vi "ep_Write Inf File.vi"(8 "error in":errorcluster, 10 "inf content":string, 11 "task in":T1={"file refnums"=[], "Data Object"=refnum, "config info"={"station_name"="", "rec_dev_id"="", "rev_year"=1999.0, "TT"=0, "##A"=0, "##D"=0, "analog channel info"=[], "status channel info"=[], "lf"=-inf, "nrates"=65535, "samp info"=[], "initial timestamp"=timestamp(0 s since 1904-01-01), "trigger timestamp"=timestamp(0 s since 1904-01-01), "ft"=enum."Binary", "timemult"=1.0}, "public inf content"={"Source"="", "Record Type"=enum."Fault", "Phase ID"="", "Event Description"="", "Device ID"="", "Distance of Fault"=-1.0, "Distance Unit"=enum."Miles", "Max_Current"=inf, "Min_Current"=-inf, "Max_Voltage"=inf, "Min_Voltage"=-inf, "EventNoteCount"=0, "Event Information"=[]}, "private inf content"=[], "internal buffers"={"start index"=1, "config to public inf"=enum."disabled", "static config info"="", "static file_des record inf"="", "static file_des channel inf"="", "public inf"="", "private inf"=""}} {"public inf content"."Event Information"."min sample number" max=9999999999; "public inf content"."Event Information"."max sample number" max=9999999999; "config info"."nrates" max=999; "config info"."status channel info"."Dn" min=1 max=999999; "config info"."analog channel info"."An" min=1 max=999999; "config info"."trigger timestamp" format="%<%H:%M:%S%6u\n%d/%m/%Y>T"; "config info"."initial timestamp" format="%<%H:%M:%S%6u\n%d/%m/%Y>T"; "config info"."##D" max=999999; "config info"."##A" max=999999; "config info"."TT" min=1 max=999999; "config info"."rev_year" min=1999.0 max=1999.0}) -> (0 "error out":errorcluster, 3 "dup task":T1={"file refnums"=[], "Data Object"=refnum, "config info"={"station_name"="", "rec_dev_id"="", "rev_year"=1999.0, "TT"=0, "##A"=0, "##D"=0, "analog channel info"=[], "status channel info"=[], "lf"=-inf, "nrates"=65535, "samp info"=[], "initial timestamp"=timestamp(0 s since 1904-01-01), "trigger timestamp"=timestamp(0 s since 1904-01-01), "ft"=enum."Binary", "timemult"=1.0}, "public inf content"={"Source"="", "Record Type"=enum."Fault", "Phase ID"="", "Event Description"="", "Device ID"="", "Distance of Fault"=-1.0, "Distance Unit"=enum."Miles", "Max_Current"=inf, "Min_Current"=-inf, "Max_Voltage"=inf, "Min_Voltage"=-inf, "EventNoteCount"=0, "Event Information"=[]}, "private inf content"=[], "internal buffers"={"start index"=1, "config to public inf"=enum."disabled", "static config info"="", "static file_des record inf"="", "static file_des channel inf"="", "public inf"="", "private inf"=""}} {"public inf content"."Event Information"."min sample number" max=9999999999; "public inf content"."Event Information"."max sample number" max=9999999999; "config info"."nrates" max=999; "config info"."status channel info"."Dn" min=1 max=999999; "config info"."analog channel info"."An" min=1 max=999999; "config info"."trigger timestamp" format="%<%H:%M:%S%6u\n%d/%m/%Y>T"; "config info"."initial timestamp" format="%<%H:%M:%S%6u\n%d/%m/%Y>T"; "config info"."##D" max=999999; "config info"."##A" max=999999; "config info"."TT" min=1 max=999999; "config info"."rev_year" min=1999.0 max=1999.0})   [LabVIEW 2011, in "NI_EP_COMTRADE.lvlib"]
uses:
  <vilib>/addons/Electrical Power/File IO/NI_EP_COMTRADE.lvlib
  <vilib>/addons/Electrical Power/File IO/COMTRADE/typedefs/ep_Task.ctl
  <vilib>/addons/Electrical Power/File IO/COMTRADE/typedefs/ep_Config Info.ctl
  <vilib>/addons/Electrical Power/File IO/COMTRADE/typedefs/ep_Analog Channel Info.ctl
  <vilib>/addons/Electrical Power/File IO/COMTRADE/typedefs/ep_Status Channel Info.ctl
  <vilib>/addons/Electrical Power/File IO/COMTRADE/typedefs/ep_File Format.ctl
  <vilib>/addons/Electrical Power/File IO/COMTRADE/typedefs/ep_Public Inf Content.ctl
  <vilib>/addons/Electrical Power/File IO/COMTRADE/typedefs/ep_Public Event Inf.ctl
  <vilib>/addons/Electrical Power/File IO/COMTRADE/typedefs/ep_Private Inf Content.ctl
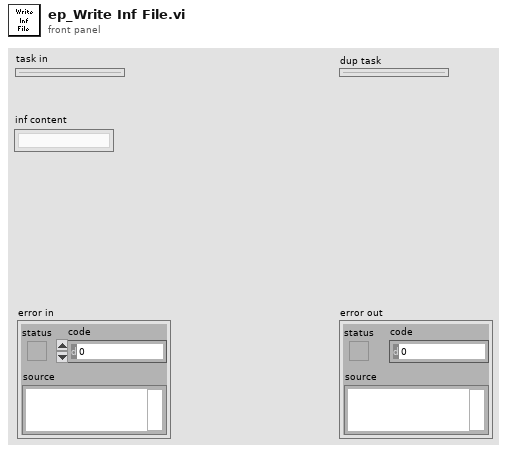
[diagram p1: front panel]
types:
  T1 = typedef "NI_EP_COMTRADE.lvlib/ep_Task.ctl" = cluster{"file refnums":refnum<file>[], "Data Object":refnum<k20>, "config info":T2, "public inf content":T6, "private inf content":T8, "internal buffers":cluster{"start index":u32, "config to public inf":enum16{"disabled", "enabled", "buffered"}, "static config info":string, "static file_des record inf":string, "static file_des channel inf":string, "public inf":string, "private inf":string}}
  T2 = typedef "NI_EP_COMTRADE.lvlib/ep_Config Info.ctl" = cluster{"station_name":string, "rec_dev_id":string, "rev_year":dbl, "TT":u32, "##A":u32, "##D":u32, "analog channel info":T3[], "status channel info":T4[], "lf":sgl, "nrates":u16, "samp info":cluster{"samp":sgl, "endsamp":u32}[], "initial timestamp":timestamp, "trigger timestamp":timestamp, "ft":T5, "timemult":sgl}
  T3 = typedef "NI_EP_COMTRADE.lvlib/ep_Analog Channel Info.ctl" = cluster{"An":u32, "ch_id":string, "ph":string, "ccbm":string, "uu":string, "a":sgl, "b":sgl, "skew":sgl, "min":i32, "max":i32, "primary":sgl, "secondary":sgl, "PS":enum16{"P", "S"}}
  T4 = typedef "NI_EP_COMTRADE.lvlib/ep_Status Channel Info.ctl" = cluster{"Dn":u32, "ch_id":string, "ph":string, "ccbm":string, "Y":bool}
  T5 = typedef "NI_EP_COMTRADE.lvlib/ep_File Format.ctl" = enum16{"ASCII", "Binary"}
  T6 = typedef "NI_EP_COMTRADE.lvlib/ep_Public Inf Content.ctl" = cluster{"Source":string, "Record Type":enum16{"Fault", "Unknown", "Misoperation", "Close", "Trip", "Reclose", "Power swing", "Simulation"}, "Phase ID":string, "Event Description":string, "Device ID":string, "Distance of Fault":dbl, "Distance Unit":enum16{"Miles", "Kilometers", "Percent of line", "Percent of setting", "Ohms"}, "Max_Current":dbl, "Min_Current":dbl, "Max_Voltage":dbl, "Min_Voltage":dbl, "EventNoteCount":u32, "Event Information":T7[]}
  T7 = typedef "NI_EP_COMTRADE.lvlib/ep_Public Event Inf.ctl" = cluster{"channel number":u32, "max value":dbl, "min value":dbl, "max sample number":u64, "min sample number":u64, "max sample text":string[], "min sample text":string[]}
  T8 = typedef "NI_EP_COMTRADE.lvlib/ep_Private Inf Content.ctl" = cluster{"Section Header":string, "Entry Names":string[], "Entry Values":string[]}[]
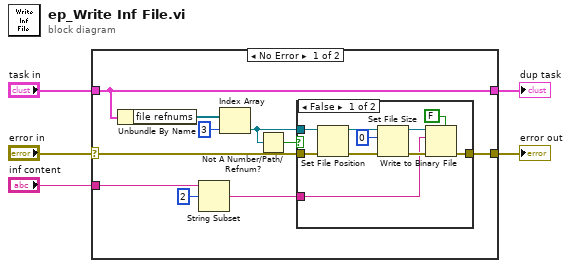
[diagram p0: block diagram]
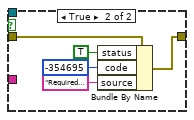
[diagram p2: hidden frame]
diagram:
  n1 = case shown="No Error" "error in" {
    selector: "error in" -> [w12 w31]
    tunnel: "task in" -> [w13 w32]
    tunnel: [w13 w32] -> w3
    tunnel: [w11 w31] -> w2
    tunnel: "inf content" -> [w10 _]
    frame No Error {
      n2 = Unbundle By Name(w13) -> ("file refnums"=w15:refnum<file>[])
      n3 = String Subset(string=w10, offset (0)=2) -> (substring=w6:string)  [unwired: 1 in]
      n4 = Index Array(array=w15, index=3) -> (element=w8:refnum<file>)
      n5 = Not A Number/Path/Refnum?(number/path/refnum=w8) -> (NaN/Path/Refnum?=w7:bool)
      n6 = case shown="False" w7 {
        tunnel: w8 -> [w22 _]
        tunnel: w12 -> [w19 w28]
        tunnel: [w18 w27] -> w11
        tunnel: w6 -> [w17 _]
        frame False {
          n7 = Set File Position(refnum=w22, error in=w19) -> (refnum out=w23:refnum<file>, error out=w25:errorcluster)  [unwired: 2 in]
          n8 = Set File Size(4:w25, 6:i64 0 ("size (in bytes)"), 7:w23) -> (0:w20:errorcluster, 3:w21:refnum<file>)
          n9 = Write to Binary File(file (use dialog)=w21, data=w17, error in=w20, 5:FALSE ("prepend array or string size? (T)")) -> (error out=w18:errorcluster)  [unwired: 2 in, 2 out]
        }
        frame True {
          n10 = Bundle By Name(cluster=w28, "status"=TRUE, "code"=-354695, "source"="Required file not opened") -> (w27:errorcluster)
        }
      }
    }
    frame Error {
    }
  }
  "dup task" <- w3
  "error out" <- w2
